vi "pid_manual_motion_v2.vi"(8 "inputValid":bool=TRUE, 9 "lastPosValid":bool=TRUE, 10 "lastPos":fxp<+/-,32,4>, 11 "manualMotion":T1) -> (0 "moving":bool, 1 "outputValid":bool, 3 "output":fxp<+/-,32,4>)   [LabVIEW 2016]
uses:
  <vilib>/rvi/FXPMathLib/FxpSub/XNode/nifxpmath_Sub.xnode
  <vilib>/rvi/FXPMathLib/FxpMul/XNode/nifxpmath_Multiplier.xnode
  <vilib>/rvi/FXPMathLib/FxpAdd/XNode/nifxpmath_Add.xnode
  <vilib>/rvi/FXPMathLib/sim/FxpSim.dll
  <instrlib>/_niInstr/Basic Elements/v1/FPGA/niInstr Basic Elements v1 FPGA.lvlib
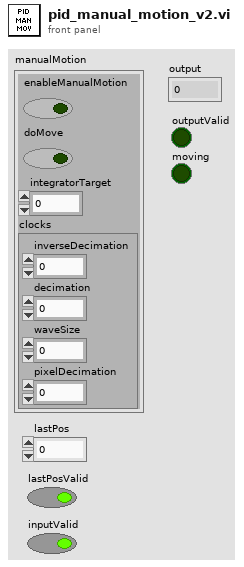
[diagram p1: front panel]
types:
  T1 = cluster{"enableManualMotion":bool, "doMove":bool, "integratorTarget":fxp<+/-,22,2>, "clocks":cluster{"inverseDecimation":fxp<+,22,0>, "decimation":u16, "waveSize":u16, "pixelDecimation":u16}}
  T2 = cluster{"inverseDecimation":fxp<+,22,0>, "decimation":u16, "waveSize":u16, "pixelDecimation":u16}
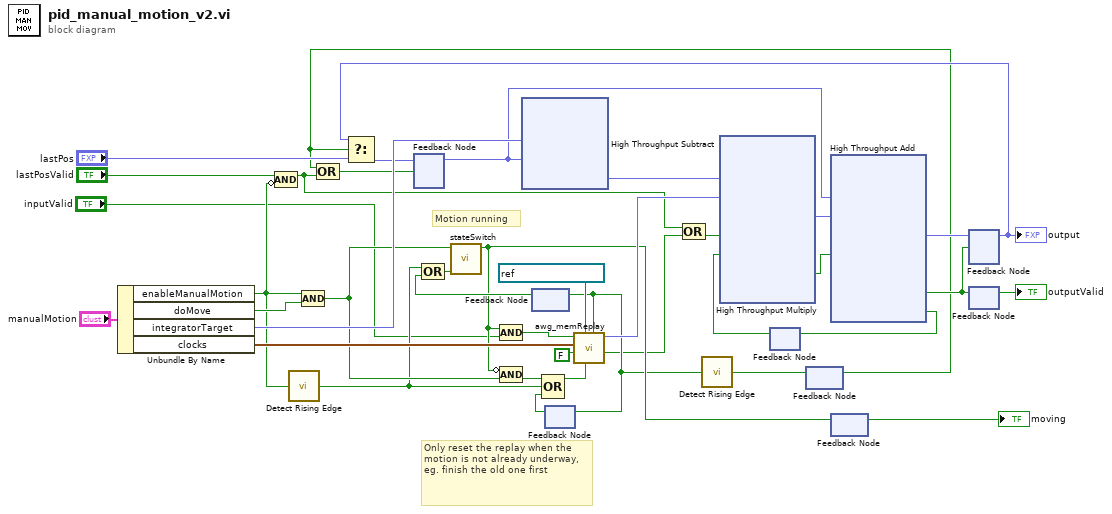
[diagram p0: block diagram]
diagram:
  # "Only reset the replay when the motion is not already underway, eg. finish the old one first"
  # "Motion running"
  n1 = Unbundle By Name("manualMotion") -> ("enableManualMotion"=w17:bool, "doMove"=w27:bool, "integratorTarget"=w38:fxp<+/-,22,2>, "clocks"=w30:T2)
  n2 = Compound Arithmetic op=AND("lastPosValid", invert w17) -> (w5:bool)
  n3 = call <instrlib>:"Detect Rising Edge.vi"("signal"=w17) -> ("edge detected"=w14:bool)  [unwired: 14 in]
  n4 = Compound Arithmetic op=AND(w17, w27) -> (w26:bool)
  n5 = feedback #1() -> (w21:fxp<+/-,32,4>)  [unwired: 1 in]
  n6 = xnode ("High Throughput Subtract")("x"=w38, "y"=w21) -> ("x-y"=w37:fxp<+/-,22,2>)
  n7 = feedback #2() -> (w15:bool)  [unwired: 1 in]
  n8 = Compound Arithmetic op=OR(w14, w15) -> (w16:bool)
  n9 = call "stateSwitch.vi"("disable"=w16, "enable"=w26) -> ("state"=w13:bool)  [unwired: 9 in]
  n10 = Compound Arithmetic op=AND(w13, "inputValid") -> (w25:bool)
  n11 = Compound Arithmetic op=AND(invert w13, w26) -> (w20:bool)
  n12 = feedback #3() -> (w12:bool)  [unwired: 1 in]
  n13 = Compound Arithmetic op=OR(w20, w14, w12) -> (w18:bool)
  n14 = call "awg_memReplay.vi"("reset"=w18, "memSelector"=refnum<k21> "fb.mot.motion", "periodic"=FALSE, "clocks"=w30, "output"=w25) -> ("outputValid"=w7:bool, "interpOutput"=w24:fxp<+/-,19,2>, "replayDone"=w8:bool)  [unwired: 2 in, 2 out]
  n15 = feedback-in #2(w8) -> ()
  n16 = feedback-in #3(w8) -> ()
  n17 = Compound Arithmetic op=OR(w5, w7) -> (w6:bool)
  n18 = call <instrlib>:"Detect Rising Edge.vi"("signal"=w8) -> ("edge detected"=w19:bool)  [unwired: 14 in]
  n19 = feedback #4() -> (w34:bool)  [unwired: 1 in]
  n20 = xnode ("High Throughput Multiply")("x"=w37, "y"=w24, "input valid"=w6, "ready for output (T)"=w34) -> ("x*y"=w33:fxp<+/-,22,2>, "output valid"=w36:bool)  [unwired: 1 out]
  n21 = feedback #5() -> (w1:bool)  [unwired: 1 in]
  n22 = Compound Arithmetic op=OR(w1, w5) -> (w22:bool)
  n23 = feedback-in #5(w19) -> ()
  n24 = xnode ("High Throughput Add")("x"=w21, "y"=w33, "input valid"=w36) -> ("x+y"=w3:fxp<+/-,32,4>, "output valid"=w9:bool, "ready for input"=w35:bool)  [unwired: 1 in]
  n25 = feedback-in #4(w35) -> ()
  n26 = feedback-in #6(w13) -> ()
  n27 = feedback #6() -> (→"moving":bool)  [unwired: 1 in]
  n28 = feedback #7() -> (w2:fxp<+/-,32,4>)  [unwired: 1 in]
  "output" <- w2
  n29 = Select(t=w2, s=w1, f="lastPos") -> (s? t:f=w23:fxp<+/-,32,4>)
  n30 = feedback-in #1(w23, w22) -> ()
  n31 = feedback-in #7(w3, w9) -> ()
  n32 = feedback #8() -> (→"outputValid":bool)  [unwired: 1 in]
  n33 = feedback-in #8(w9) -> ()
